vi "Set_Exe_Data.vi"(8 "error in (no error)":errorcluster, 10 "data":T1, 11 "Class in":refnum<class "AB_EXE.lvclass">) -> (0 "error out":errorcluster, 3 "Class out":refnum<class "AB_EXE.lvclass">)   [LabVIEW 2020, in "AB_EXE.lvclass"]
uses:
  <vilib>/AppBuilder/AB_Classes/EXE/AB_EXE.lvclass
  <vilib>/AppBuilder/AB_Classes/EXE/AB_EXE.ctl
  <vilib>/AppBuilder/AB_Classes/EXE/AB_EXE_SharedVar_Deploy.ctl
  <vilib>/AppBuilder/AB_Classes/EXE/AB_EXE_SharedVar_LibInfo.ctl
  <vilib>/AppBuilder/AB_Classes/EXE/AB_EXE.lvclass/AB_EXE.ctl
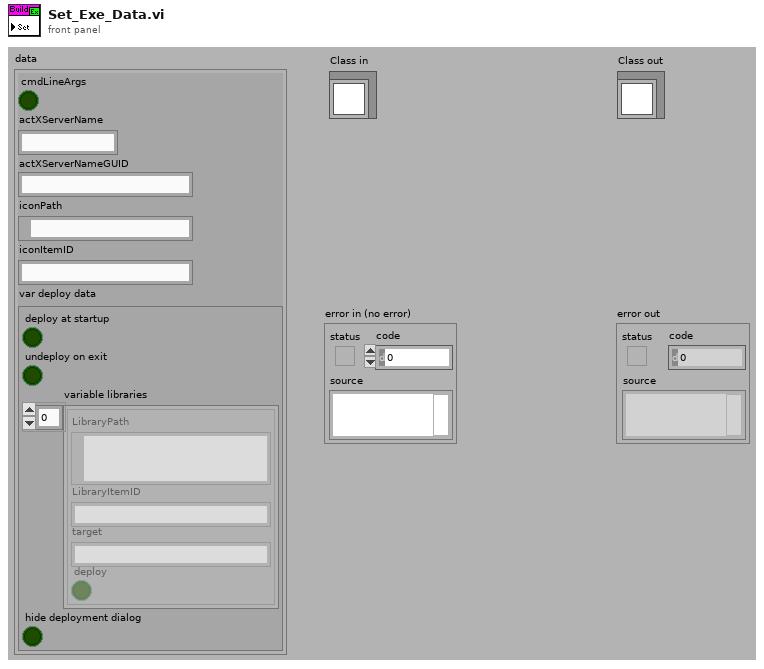
[diagram p1: front panel]
types:
  T1 = typedef "AB_EXE.ctl" = cluster{"cmdLineArgs":bool, "actXServerName":string, "actXServerNameGUID":string, "iconPath":path, "iconItemID":string, "var deploy data":T2}
  T2 = typedef "AB_EXE_SharedVar_Deploy.ctl" = cluster{"deploy at startup":bool, "undeploy on exit":bool, "variable libraries":T3[], "hide deployment dialog":bool}
  T3 = typedef "AB_EXE_SharedVar_LibInfo.ctl" = cluster{"LibraryPath":path, "LibraryItemID":string, "target":string, "deploy":bool}
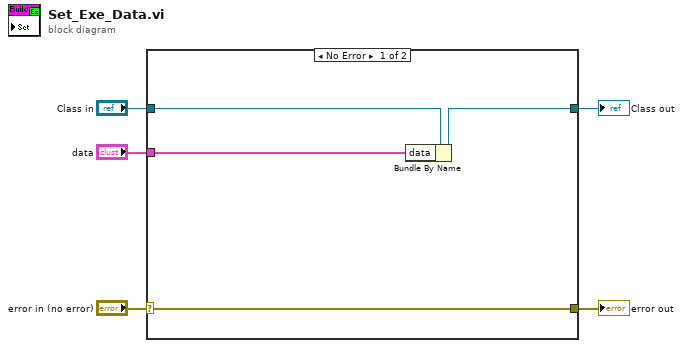
[diagram p0: block diagram]
diagram:
  n1 = case "Case" shown="No Error" "error in (no error)" {
    selector: "error in (no error)" -> [w9 w11]
    tunnel: [w9 w11] -> w4
    tunnel: [w8 w10] -> w2
    tunnel: "Class in" -> [w7 w10]
    tunnel: "data" -> [w6 _]
    frame No Error {
      n2 = Bundle By Name(cluster=w7, "data"=w6) -> (w8:refnum<class "AB_EXE.lvclass">)
    }
    frame Error {
    }
  }
  "error out" <- w4
  "Class out" <- w2
